vi "Loader.vi"(0 "Enum":enum16{"Start", "Run", "End"}(ring), 1 "Run":bool) -> ()   [LabVIEW 2012]
uses:
  TypeDefs/PWM Module 1.ctl
  <vilib>/Rock Robotics/SystemInterfaces/Typedef/FPGA_TypedefDigitalModule.ctl
  <vilib>/Rock Robotics/SystemInterfaces/DIO/FPGA_DIOPWMChannel.ctl
  <vilib>/Rock Robotics/SystemInterfaces/DIO/FPGA_DIORelayChannel.ctl
  <vilib>/Rock Robotics/WPI/Relay/WPI_RelayValue.ctl
panel:
  in  "PWM Module (DIO A)":T1={"Module"=enum."Digital Module 1", "Shooter"=enum."PWM 1", "Right Drive"=enum."PWM 2", "Arm"=enum."PWM 3", "Left Drive"=enum."PWM 4", "Compress"=enum."PWM 5", "Arm Servo"=enum."PWM 6", "Unassigned"=enum."PWM 7", "Unassigned"=enum."PWM 8", "Unassigned"=enum."PWM 9", "Unassigned"=enum."PWM 10", "Loader"=enum."Relay 1", "Compressor"=enum."Relay 2", "Unassigned"=enum."Relay 3", "Unassigned"=enum."Relay 4", "Unassigned"=enum."Relay 5", "Unassigned"=enum."Relay 6", "Unassigned"=enum."Relay 7", "Unassigned "=enum."Relay 8"}
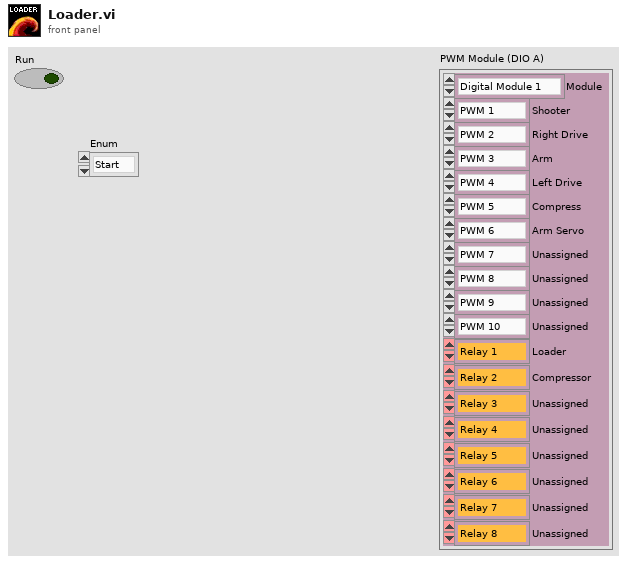
[diagram p1: front panel]
types:
  T1 = typedef "PWM Module 1.ctl" = cluster{"Module":T2, "Shooter":T3, "Right Drive":T3, "Arm":T3, "Left Drive":T3, "Compress":T3, "Arm Servo":T3, "Unassigned":T3, "Unassigned":T3, "Unassigned":T3, "Unassigned":T3, "Loader":T4, "Compressor":T4, "Unassigned":T4, "Unassigned":T4, "Unassigned":T4, "Unassigned":T4, "Unassigned":T4, "Unassigned ":T4}
  T2 = typedef "FPGA_TypedefDigitalModule.ctl" = enum16{"Digital Module 1", "Digital Module 2"}
  T3 = typedef "FPGA_DIOPWMChannel.ctl" = enum8{"PWM 1", "PWM 2", "PWM 3", "PWM 4", "PWM 5", "PWM 6", "PWM 7", "PWM 8", "PWM 9", "PWM 10", "Invalid"}
  T4 = typedef "FPGA_DIORelayChannel.ctl" = enum8{"Relay 1", "Relay 2", "Relay 3", "Relay 4", "Relay 5", "Relay 6", "Relay 7", "Relay 8", "Invalid"}
  T5 = typedef "WPI_RelayValue.ctl" = enum16{"Off", "On", "Forward", "Reverse"}
  T6 = typedef "WPI_RelayDevRef.ctl" = cluster{"DevStatus":errorcluster, "Relay Channel":T4, "Digital Module":T2, "Relay Direction":T7}
  T7 = typedef "WPI_RelayDirection.ctl" = enum16{"Both directions", "Forward only", "Reverse only"}
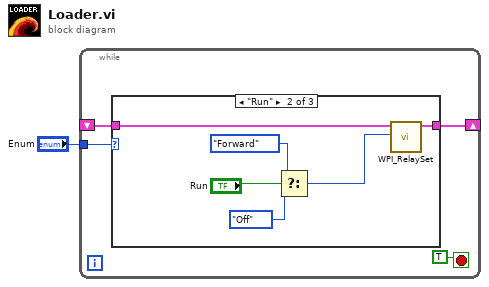
[diagram p0: block diagram]
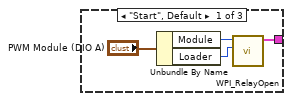
[diagram p2: hidden frame]
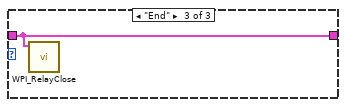
[diagram p3: hidden frame]
diagram:
  n1 = while {
    shift-right: [w5] -> _
    shift-left: _ -> [w4]
    tunnel: "Enum" -> [w2]
    stop <- TRUE stop-if-true
    n2 = case shown="\"Run\"" w2 {
      tunnel: [w8 w14 w16] -> w5
      tunnel: w4 -> [_ w15 w16]
      frame "Start", Default {
        n3 = Unbundle By Name("PWM Module (DIO A)") -> ("Module"=w9:T2, "Loader"=w6:T4)
        n4 = call <vilib>:"WPI_RelayOpen.vi"("Relay Channel"=w6, "Digital Module (Module 1)"=w9) -> ("RelayDevRef"=w8:T6)  [unwired: 8 in, 1 out]
      }
      frame "Run" {
        n5 = Select(t=WPI_RelayValue."Forward" ("RelayValue"), s="Run", f=WPI_RelayValue."Off" ("RelayValue")) -> (s? t:f=w10:T5)
        n6 = call <vilib>:"WPI_RelaySet.vi"("RelayValue"=w10, "RelayDevRef"=w15) -> ("RelayDevRef"=w14:T6)  [unwired: 8 in, 1 out]
      }
      frame "End" {
        n7 = call <vilib>:"WPI_RelayClose.vi"("RelayDevRef"=w16) -> ()  [unwired: 10 in, 1 out]
      }
    }
  }
